vi "RMFlush.vi"(8 "error in (no error)":errorcluster, 11 "ResultManager":T1={"InstancePtr"=0, "ResultManagerConfig"={"Number of beads"=0, "Number of frame info columns"=0, "Result scaling"={"X"=0.0, "Y"=0.0, "Z"=0.0}, "Result offset"={"X"=0.0, "Y"=0.0, "Z"=0.0}, "Write Interval"=100, "Max frames in memory"=100, "Binary output (1/0)"=0}}) -> (0 "error":errorcluster, 3 "ResultManager (out)":T1={"InstancePtr"=0, "ResultManagerConfig"={"Number of beads"=0, "Number of frame info columns"=0, "Result scaling"={"X"=0.0, "Y"=0.0, "Z"=0.0}, "Result offset"={"X"=0.0, "Y"=0.0, "Z"=0.0}, "Write Interval"=100, "Max frames in memory"=100, "Binary output (1/0)"=0}})   [LabVIEW 2011]
uses:
  ResultManagerInstance.ctl
  ResultManagerConfig.ctl
  XYZf.ctl
  QTrkDLL.vi
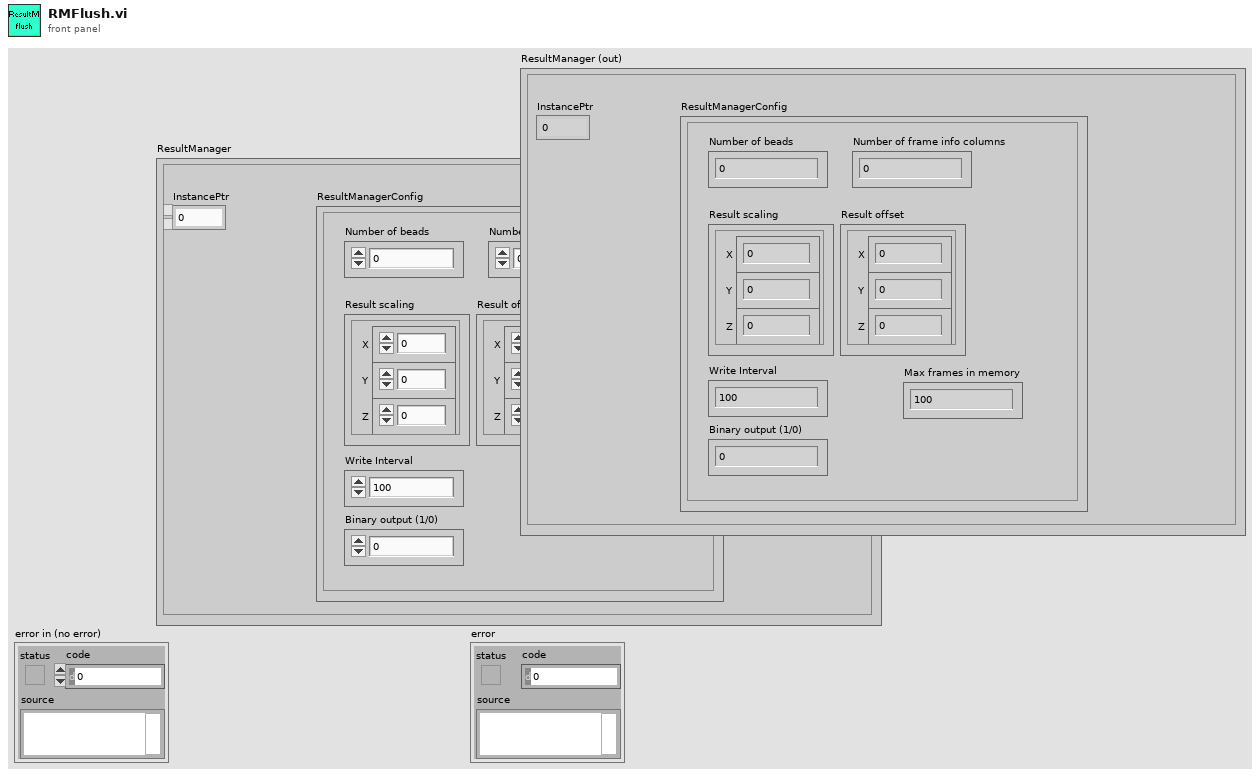
[diagram p1: front panel]
types:
  T1 = typedef "ResultManagerInstance.ctl" = cluster{"InstancePtr":u64, "ResultManagerConfig":T2}
  T2 = typedef "ResultManagerConfig.ctl" = cluster{"Number of beads":i32, "Number of frame info columns":i32, "Result scaling":T3, "Result offset":T3, "Write Interval":i32, "Max frames in memory":i32, "Binary output (1/0)":i8}
  T3 = typedef "XYZf.ctl" = cluster{"X":sgl, "Y":sgl, "Z":sgl}
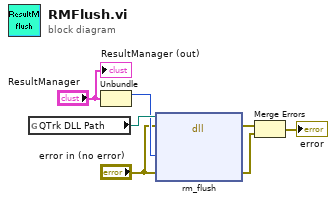
[diagram p0: block diagram]
diagram:
  n1 = global read "QTrkDLL.vi" "QTrk DLL Path"() -> (w7:path)
  n2 = Unbundle("ResultManager") -> ("InstancePtr"=w5:u64)  [unwired: 1 out]
  n3 = dll-call lib="D:/jcnossen1/cudaqi-tracker/bin/jtrk-labview.dll" fn="rm_flush"(path in=w7, error in="error in (no error)", "resultmanager"=w5, "error"="error in (no error)") -> (error out=w3:errorcluster, "error"=w2:errorcluster)  [unwired: 3 in, 1 out]
  n4 = Merge Errors(w3, w2) -> (→"error":errorcluster)
  "ResultManager (out)" <- "ResultManager"
